vi "WBA 256 Sector (FPGA-SIM).vi"() -> ()   [LabVIEW 2013]
doc: "This is the FPGA VI for the 10-Tap 8-Bit Camera with DRAM example. This example demonstrates how to acquire images from a 10-tap, 8-bit, extended configuration, Camera Link camera and transfer the images to the host. This example supports area scan and line scan cameras for both continuous and finite acquisitions.\n\nThis example also demonstrates the use of DRAM as a frame buffer for very high speed acquisitions. Data packing and flow-control are also employed to maximize use of the available DRAM and FIFOs in terms of both memory space and performance.\n\nAdditionally, the example demonstrates the serial server, which allows third-party camera configuration utilities to communicate with the camera using the Camera Link serial interface while this VI is running."
uses:
  Common/CL Signal Mapping.ctl
  Common/CL Configuration.ctl
  FPGA/Sector/Accumulate/Sector Parameter Cluster.ctl
  <vilib>/Platform/TimedLoop/XDataNode/timing_clust.ctl
  <vilib>/Platform/TimedLoop/XDataNode/nitl_modes.ctl
  <vilib>/Platform/TimedLoop/XDataNode/wakeup.ctl
  <vilib>/rvi/Emulation/niFpgaSctlEmulationGetInTimedLoop.vi
  <vilib>/rvi/Emulation/niFpgaEmulationReportErrorSimple.vi
  <vilib>/rvi/Emulation/niFpgaGetClockAttributes.vi
  <vilib>/rvi/Emulation/niFpgaCriticalErrorInLSC.vi
  FPGA/Globals/Accumulated Sector Intensity.vi
  <vilib>/rvi/FIFO/Fifo_Resource/nirvififoEmulationGetNumberOfElementsToWriteFpgaImpl.vi
  <vilib>/rvi/DataTransferAndStorage/Container/Common/niFpgaContainerGetUniqueNameForEmu.vi
  <vilib>/rvi/interface/RandomDataEmulation/nirviRandomDataFPGAFIFO.vi
  <vilib>/rvi/interface/RandomDataEmulation/niFpgaRandomDataHandleErrors.vi
  <vilib>/rvi/FIFO/Fifo_Resource/nirvififoEmulationWriteFpgaImpl.vi
  <vilib>/rvi/FIFO/Fifo_Resource/nirvififoEmulationGetNumberOfElementsToReadFpgaImpl.vi
  <vilib>/rvi/FIFO/Fifo_Resource/nirvififoEmulationReadFpgaImpl.vi
  <vilib>/rvi/Emulation/niFpgaProcessEmulError.vi
  FPGA/Globals/Sector Parameter Global.vi
  <vilib>/rvi/eio/common/nirviEmuTemplateMethod_errors.vi
  FPGA/Globals/Pixel Location Global.vi
  <vilib>/Platform/TimedLoop/XDataNode/XDataNode.xnode
  <vilib>/rvi/DataTransferAndStorage/Container/XNode/niFpgaContainer.xnode
  <vilib>/rvi/FIFO/Fifo_Resource/nirvififoEmulationGetNumberOfElementsToWrite.vi
  <vilib>/rvi/interface/RandomDataEmulation/nirviRandomDataFpgaReadWriteTemplate.vi
  <vilib>/rvi/FIFO/Fifo_Resource/nirvififoEmulationWrite.vi
  <vilib>/rvi/FIFO/Fifo_Resource/nirvififoEmulationGetNumberOfElementsToRead.vi
  <vilib>/rvi/FIFO/Fifo_Resource/nirvififoEmulationRead.vi
  <vilib>/eio/EIONode/EIONode.xnode
  <vilib>/Platform/TimedLoop/XDataNode/XDNodeRunTimeDep.lvlib
panel:
  out "Left Sector Edge":u8
  out "Right Sector Edge":u8
  in  "Right Start Angle Duty Cycle":fxp<+,8,0>
  in  "Right End Angle Duty Cycle":fxp<+,8,0>
  in  "Left End Angle Duty Cycle":fxp<+,8,0>
  in  "Left Start Angle Duty Cycle":fxp<+,8,0>
  out "Number of Elements to Write Sector Grouping FIFO":u32
  out "Analysis Ticks":u32
  out "Target Sim TO":bool
  out "Cam Data Timeout":bool
  out "Sector FIFO Timeout":bool
  out "Host DMA Timeout":bool
  out "Number of Elements to Read Cam Data":u32
  out "Number of Elements to Write Host DMA":u32
  in  "Words per image":u32=1000
  in  "Y Resolution":u16=1000
  in  "X Resolution":u16=1000
  in  "[Average BG Intensity]":u8[](array[numeric])=[0, 0, 0, 0, 0, 0, 0, 0, 0, 0, 0, 0, 0, 0, 0, 0, 0, 0, 0, 0, 0, 0, 0, 0, 0, 0, 0, 0, 0, 0, 0, 0]
  in  "Sector Threshold":u8
  in  "# of Frames to Average":u8=1
  in  "Sector Parameters Right":T1={"Start Angle"=0.0, "End Angle"=0.4708251953125, "Inner Radius"=309, "Outter Radius"=405, "Hinge X"=685, "Hinge Y"=527, "NumWingSectors"=8}
  in  "Sector Parameters Left":T1={"Start Angle"=0.65740966796875, "End Angle"=0.99468994140625, "Inner Radius"=309, "Outter Radius"=405, "Hinge X"=464, "Hinge Y"=534, "NumWingSectors"=8}
  in  "CL Config.Configuration":T2=enum."Full"
  in  "CL Config.Signal Mapping":T3=enum."Basler 10-tap"
  in  "CL Config.Line Scan":bool
  in  "CL Config.DVAL Active High":bool=TRUE
  in  "CL Config.LVAL Active High":bool=TRUE
  in  "CL Config.FVAL Active High":bool=TRUE
  in  "CL Config.Spare Active High":bool=TRUE
  in  "Acq Control.Line Scan Height":u32
  in  "Acq Control.Frames To Acq":u32
  in  "Acq Control.Acquire":bool
  in  "Acq Control.Cancel Acq":bool
  in  "Acq Control.Ignore DVAL":bool
  in  "Acq Control.Initialize":bool
  out "Acq Status.Acq In Progress":bool
  out "Acq Status.Clocks Per Line":u32
  out "Acq Status.Frames Acq'd":u32
  out "Acq Status.Lines Per Frame":u32
  out "Acq Status.DMA Write Timeout":bool
  out "Acq Status.Initialized":bool
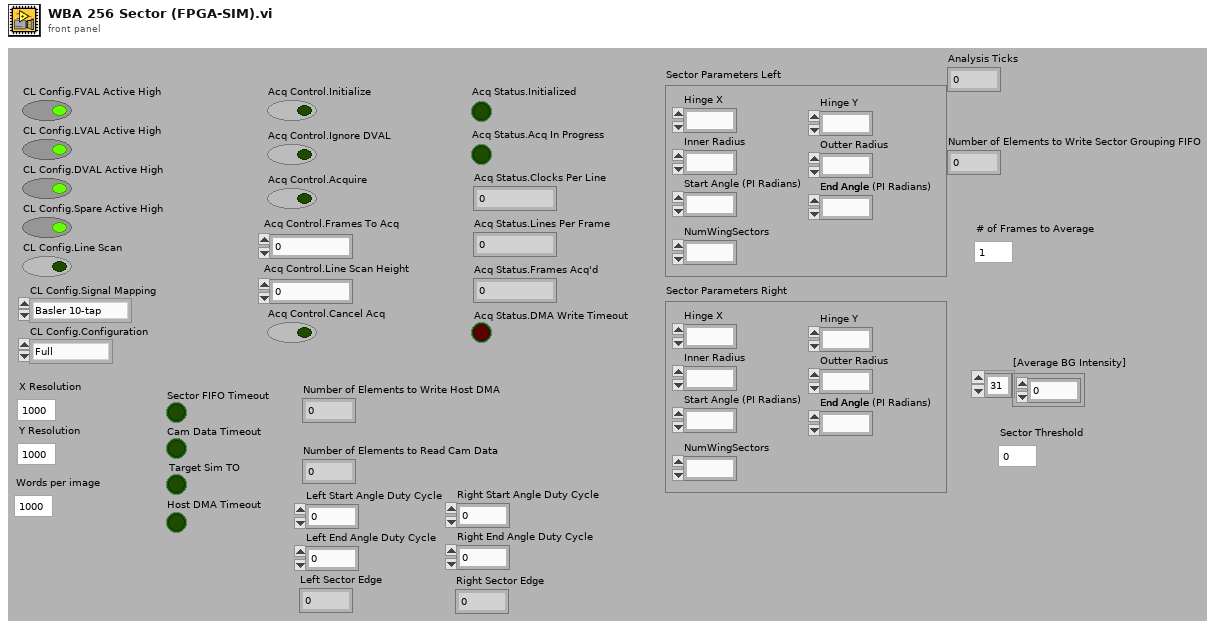
[diagram p1: front panel]
types:
  T1 = typedef "Sector Parameter Cluster.ctl" = cluster{"Start Angle":fxp<+/-,17,2>, "End Angle":fxp<+/-,17,2>, "Inner Radius":u16, "Outter Radius":u16, "Hinge X":u16, "Hinge Y":u16, "NumWingSectors":u8}
  T2 = typedef "CL Configuration.ctl" = enum8{"Base", "Medium", "Full"}
  T3 = typedef "CL Signal Mapping.ctl" = enum8{"Standard", "Basler 10-tap", "Vosskühler 10-tap"}
  T4 = typedef "XDNodeRunTimeDep.lvlib/timing_clust.ctl" = cluster{"Expected End [f-1]":u64, "Actual End [f-1]":u64, "Finished Late? [f-1]":bool, "Expected End [i-1]":u64, "Actual End [i-1]":u64, "Finished Late? [i-1]":bool, "Expected Start [i]":u64, "Actual Start [i]":u64, "Expected Start [f]":u64, "Actual Start [f]":u64, "Source Name":string, "Structure Name":string, "Period":i64, "Deadline":i64, "Offset":i64, "Start":i64, "Priority":i32, "Timeout":i32, "Mode":T5, "Wakeup Reason":T6, "Error":errorcluster, "Source Type":string, "Secondary Source Type":string, "Global End Time":u64, "Global Start Time":u64, "Frame Duration":u64, "Iteration Duration":u64, "Assigned CPU":i32, "I/O Scan Engine Mode":u32}
  T5 = typedef "XDNodeRunTimeDep.lvlib/nitl_modes.ctl" = enum32{"No Change", "Process missed periods, maintain original phase", "Discard missed periods, maintain original phase", "Process missed periods, ignore original phase", "Discard missed periods, ignore original phase"}
  T6 = typedef "XDNodeRunTimeDep.lvlib/wakeup.ctl" = enum32{"Normal", "Aborted", "Asynchronous wakeup", "Timing source error", "Timed loop error", "Timeout"}
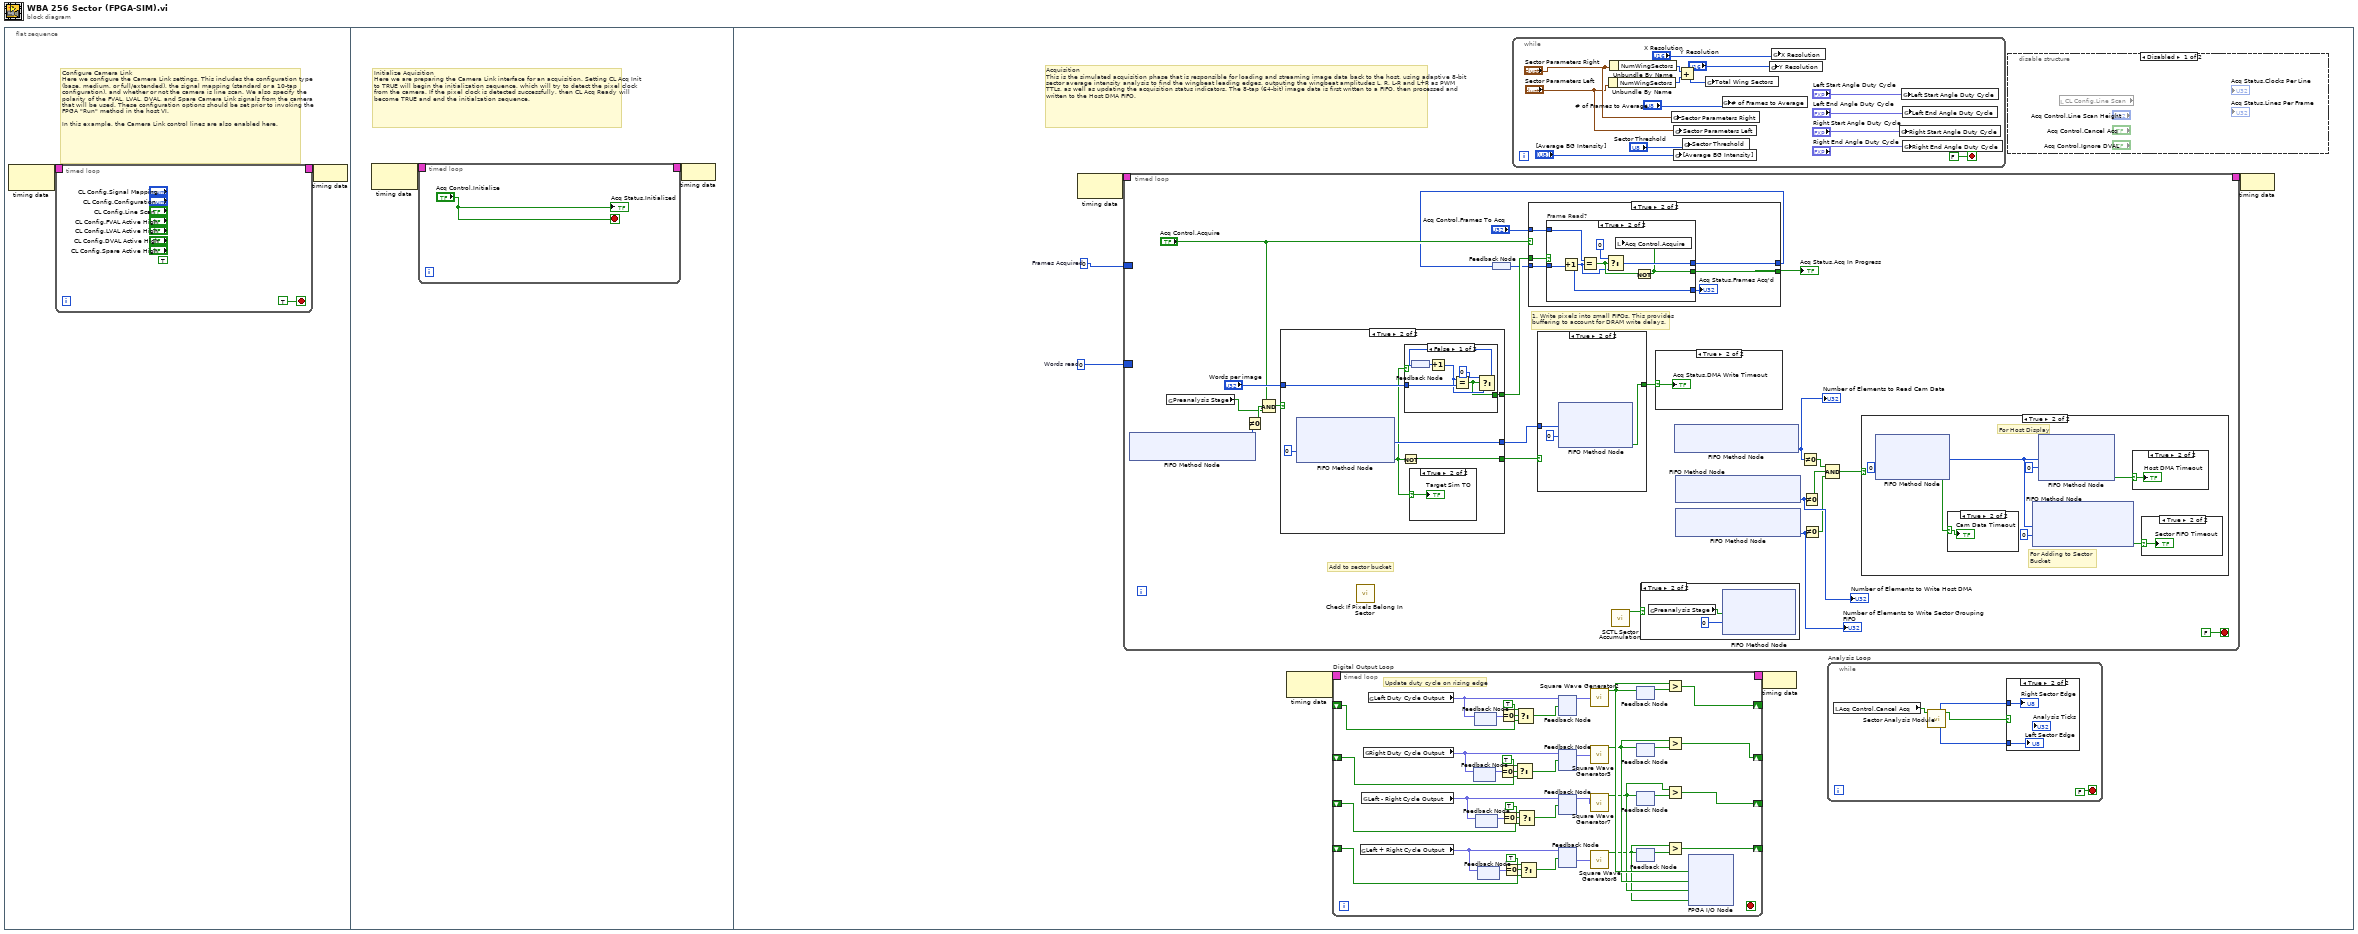
[diagram p0: block diagram]
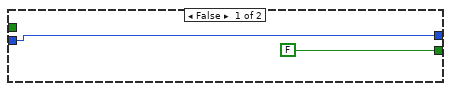
[diagram p6: hidden frame]
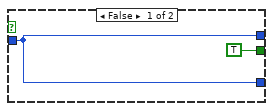
[diagram p7: hidden frame]
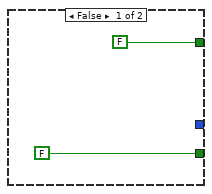
[diagram p8: hidden frame]
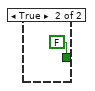
[diagram p10: hidden frame]
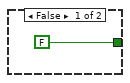
[diagram p15: hidden frame]
diagram:
  n1 = flat-sequence {
    frame #0 {
      # "Configure Camera Link\nHere we configure the Camera Link settings. This includes the configuration type (base, medium, or full/extended), the signal mapping (standard or a 10-tap configuration), and whether or not the camera is line scan. We also specify the polarity of the FVAL, LVAL, DVAL, and Spare Camera Link signals from the camera that will be used. These configuration options should be set prior to invoking the FPGA \"Run\" method in the host VI.\n\nIn this example, the Camera Link control lines are also enabled here."
      n2 = node-c288() -> (w2:T4)  [unwired: 1 in]
      n3 = timed-loop {
        timing: w2 -> [_]
        timing-out: [_] -> w1
        stop <- TRUE stop-if-true
        (unwired) TRUE ("IO Module\\CL Control Enable")
      }
      n4 = node-c288(w1) -> ()
    }
    frame #1 {
      # "Initialize Aquisition\nHere we are preparing the Camera Link interface for an acquisition. Setting CL Acq Init to TRUE will begin the initialization sequence, which will try to detect the pixel clock from the camera. If the pixel clock is detected successfully, then CL Acq Ready will become TRUE and end the initialzation sequence."
      n5 = node-c288() -> (w9:T4)  [unwired: 1 out]
      n6 = timed-loop {
        timing: w9 -> [_]
        timing-out: [_] -> w8
        stop <- "Acq Control.Initialize" stop-if-true
        "Acq Status.Initialized" <- "Acq Control.Initialize"
      }
      n7 = node-c288(w8) -> ()
    }
    frame #2 {
      w17 = u32 0  # Frames Acquired
      w18 = u32 0  # Words read
      # "Acquisition\nThis is the simulated acquisition phase that is responsible for loading and streaming image data back to the host, using adaptive 8-bit sector average intensity analysis to find the wingbeat leading edges, outputing the wingbeat amplitudes L, R, L-R and L+R as PWM TTLs, as well as updating the acquisition status indicators. The 8-tap (64-bit) image data is first written to a FIFO, then processed and written to the Host DMA FIFO."
      n8 = node-c288() -> (w20:T4)  [unwired: 1 in]
      n9 = timed-loop {
        timing: w20 -> [_]
        timing-out: [_] -> w19
        border: w18 -> [_]
        border: w17 -> [_]
        stop <- FALSE stop-if-true
        # "Add to sector bucket"
        # "1. Write pixels into small FIFOs. This provides\nbuffering to account for DRAM write delays."
        n10 = xnode ("FIFO Method Node")() -> ("Number of Elements to Write"=w88:u32)  [unwired: 1 in, 1 out]
        n11 = global read "Accumulated Sector Intensity.vi" "Preanalysis Stage"() -> (w77:bool)
        n12 = Not Equal To 0?(x=w88) -> (x != 0?=w87:bool)
        n13 = Compound Arithmetic op=AND("Acq Control.Acquire", w87, w77) -> (w95:bool)
        n14 = case shown="True" w95 {
          tunnel: [_ w127] -> w99
          tunnel: [FALSE w123] -> w97
          tunnel: "Words per image" -> [_ w125]
          tunnel: [FALSE w124] -> w84
          frame False {
          }
          frame True {
            n15 = xnode ("FIFO Method Node")("Timeout"=0) -> ("Element"=w127:u64, "Timed Out?"=w122:bool)  [unwired: 1 in, 1 out]
            n16 = Not(x=w122) -> (.not. x?=w123:bool)
            n17 = case shown="False" w122 {
              tunnel: w125 -> [w134 _]
              tunnel: [w129 FALSE] -> w124
              frame False {
                n18 = feedback #1() -> (w133:u32)
                n19 = Increment(x=w133) -> (x+1=w130:u32)
                n20 = Equal?(x=w130, y=w134) -> (x = y?=w129:bool)
                n21 = Select(t=u32 0 ("Acq Status.Frames Acq'd"), s=w129, f=w130) -> (s? t:f=w131:u32)
                n22 = feedback-in #1(w131) -> ()
              }
              frame True {
              }
            }
            n23 = case shown="True" w122 {
              selector: w122 -> [_ w128]
              frame False {
              }
              frame True {
                "Target Sim TO" <- w128
              }
            }
          }
        }
        n24 = call "Check If Pixels Belong In Sector.vi"() -> ()  [unwired: 11 in, 1 out]
        n25 = feedback #2() -> (w83:u32)
        n26 = case shown="True" "Acq Control.Acquire" {
          tunnel: w84 -> [_ w110]
          tunnel: w83 -> [w104 w109]
          tunnel: "Acq Control.Frames To Acq" -> [_ w108]
          tunnel: [w104 w107] -> w81
          tunnel: [FALSE w106] -> w80
          frame False {
          }
          frame True {
            n27 = case "Frame Read?" shown="True" w110 {
              tunnel: w109 -> [w111 w119]
              tunnel: w108 -> [_ w118]
              tunnel: [w111 w116] -> w107
              tunnel: [TRUE w114] -> w106
              tunnel: [w111 w113] -> w105
              frame False {
              }
              frame True {
                n28 = Increment(x=w119) -> (x+1=w113:u32)
                n29 = Equal?(x=w118, y=w113) -> (x = y?=w115:bool)
                n30 = Select(t=u32 0 ("Frames Acquired"), s=w115, f=w113) -> (s? t:f=w116:u32)
                n31 = Not(x=w115) -> (.not. x?=w114:bool)
                n32 = local write "Acq Control.Acquire"(w114) -> ()
              }
            }
            "Acq Status.Frames Acq'd" <- w105
          }
        }
        "Acq Status.Acq In Progress" <- w80
        n33 = feedback-in #2(w81) -> ()
        n34 = case shown="True" w97 {
          tunnel: [FALSE ("Timed Out?") w148] -> w79
          tunnel: w99 -> [_ w149]
          frame False {
          }
          frame True {
            n35 = xnode ("FIFO Method Node")("Element"=w149, "Timeout"=0) -> ("Timed Out?"=w148:bool)  [unwired: 1 in, 1 out]
          }
        }
        n36 = call "SCTL Sector Accumulation.vi"() -> ("New Data?"=w78:bool)  [unwired: 10 in, 1 out]
        n37 = case shown="True" w78 {
          frame False {
          }
          frame True {
            n38 = global read "Accumulated Sector Intensity.vi" "Preanalysis Stage"() -> (w100:bool)
            n39 = xnode ("FIFO Method Node")("Element"=w100, "Timeout"=0) -> ()  [unwired: 1 in, 2 out]
          }
        }
        n40 = case shown="True" w79 {
          selector: w79 -> [_ w102]
          frame False {
          }
          frame True {
            "Acq Status.DMA Write Timeout" <- w102
          }
        }
        n41 = xnode ("FIFO Method Node")() -> ("Number of Elements to Read"=w90:u32)  [unwired: 1 in, 1 out]
        "Number of Elements to Read Cam Data" <- w90
        n42 = xnode ("FIFO Method Node")() -> ("Number of Elements to Write"=w93:u32)  [unwired: 1 in, 1 out]
        "Number of Elements to Write Host DMA" <- w93
        n43 = xnode ("FIFO Method Node")() -> ("Number of Elements to Write"=w92:u32)  [unwired: 1 in, 1 out]
        "Number of Elements to Write Sector Grouping FIFO" <- w92
        n44 = Not Equal To 0?(x=w90) -> (x != 0?=w89:bool)
        n45 = Not Equal To 0?(x=w93) -> (x != 0?=w94:bool)
        n46 = Not Equal To 0?(x=w92) -> (x != 0?=w91:bool)
        n47 = Compound Arithmetic op=AND(w89, w94, w91) -> (w96:bool)
        n48 = case shown="True" w96 {
          frame False {
          }
          frame True {
            # "For Adding to Sector \nBucket"
            # "For Host Display"
            n49 = xnode ("FIFO Method Node")("Timeout"=0) -> ("Element"=w140:u64, "Timed Out?"=w136:bool)  [unwired: 1 in, 1 out]
            n50 = case shown="True" w136 {
              selector: w136 -> [_ w143]
              frame False {
              }
              frame True {
                "Cam Data Timeout" <- w143
              }
            }
            n51 = xnode ("FIFO Method Node")("Element"=w140, "Timeout"=0) -> ("Timed Out?"=w138:bool)  [unwired: 1 in, 1 out]
            n52 = xnode ("FIFO Method Node")("Element"=w140, "Timeout"=0) -> ("Timed Out?"=w137:bool)  [unwired: 1 in, 1 out]
            n53 = case shown="True" w137 {
              selector: w137 -> [_ w144]
              frame False {
              }
              frame True {
                "Host DMA Timeout" <- w144
              }
            }
            n54 = case shown="True" w138 {
              selector: w138 -> [_ w145]
              frame False {
              }
              frame True {
                "Sector FIFO Timeout" <- w145
              }
            }
          }
        }
      }
      n55 = node-c288() -> (w16:T4)  [unwired: 1 in]
      n56 = timed-loop "Digital Output Loop" {
        timing: w16 -> [_]
        timing-out: [_] -> w15
        shift-right: [w54] -> _
        shift-left: _ -> [w39]
        shift-right: [w53] -> _
        shift-left: _ -> [w25]
        shift-right: [w52] -> _
        shift-left: _ -> [w23]
        shift-right: [w46] -> _
        shift-left: _ -> [w21]
        stop <- _ stop-if-true
        # "Update duty cycle on rising edge"
        n57 = global read "Sector Parameter Global.vi" "Left + Right Cycle Output"() -> (w27:fxp<+,8,0>)
        n58 = global read "Sector Parameter Global.vi" "Left - Right Cycle Output"() -> (w28:fxp<+,8,0>)
        n59 = global read "Sector Parameter Global.vi" "Right Duty Cycle Output"() -> (w29:fxp<+/-,9,1>)
        n60 = global read "Sector Parameter Global.vi" "Left Duty Cycle Output"() -> (w42:fxp<+/-,9,1>)
        n61 = feedback #3() -> (w36:fxp<+/-,9,1>)  [unwired: 1 in]
        n62 = feedback-in #3(w29) -> ()
        n63 = feedback #4() -> (w41:fxp<+/-,9,1>)  [unwired: 1 in]
        n64 = feedback-in #4(w42) -> ()
        n65 = feedback #5() -> (w33:fxp<+,8,0>)  [unwired: 1 in]
        n66 = feedback-in #5(w28) -> ()
        n67 = feedback #6() -> (w30:fxp<+,8,0>)  [unwired: 1 in]
        n68 = feedback-in #6(w27) -> ()
        n69 = Equal To 0?(x=w36) -> (x = 0?=w37:bool)
        n70 = Equal To 0?(x=w41) -> (x = 0?=w43:bool)
        n71 = Equal To 0?(x=w33) -> (x = 0?=w34:bool)
        n72 = Equal To 0?(x=w30) -> (x = 0?=w31:bool)
        n73 = Select(t=TRUE, s=w37, f=w25) -> (s? t:f=w26:bool)
        n74 = Select(t=TRUE, s=w43, f=w39) -> (s? t:f=w40:bool)
        n75 = Select(t=TRUE, s=w34, f=w23) -> (s? t:f=w24:bool)
        n76 = Select(t=TRUE, s=w31, f=w21) -> (s? t:f=w22:bool)
        n77 = feedback-in #7(w42, w40) -> ()
        n78 = feedback #7() -> (w60:fxp<+/-,9,1>)  [unwired: 1 in]
        n79 = feedback #8() -> (w59:fxp<+/-,9,1>)  [unwired: 1 in]
        n80 = feedback-in #8(w29, w26) -> ()
        n81 = feedback #9() -> (w58:fxp<+,8,0>)  [unwired: 1 in]
        n82 = feedback-in #9(w28, w24) -> ()
        n83 = feedback #10() -> (w48:fxp<+,8,0>)  [unwired: 1 in]
        n84 = feedback-in #10(w27, w22) -> ()
        n85 = call "Square Wave Generator2"("duty cycle (periods)"=w60) -> ("square wave out"=w51:bool)  [unwired: 14 in]
        n86 = call "Square Wave Generator3"("duty cycle (periods)"=w59) -> ("square wave out"=w50:bool)  [unwired: 14 in]
        n87 = call "Square Wave Generator7"("duty cycle (periods)"=w58) -> ("square wave out"=w49:bool)  [unwired: 14 in]
        n88 = call "Square Wave Generator8"("duty cycle (periods)"=w48) -> ("square wave out"=w45:bool)  [unwired: 14 in]
        n89 = feedback-in #11(w51) -> ()
        n90 = feedback #11() -> (w57:bool)  [unwired: 1 in]
        n91 = feedback #12() -> (w56:bool)  [unwired: 1 in]
        n92 = feedback-in #12(w50) -> ()
        n93 = feedback #13() -> (w55:bool)  [unwired: 1 in]
        n94 = feedback-in #13(w49) -> ()
        n95 = feedback #14() -> (w47:bool)  [unwired: 1 in]
        n96 = feedback-in #14(w45) -> ()
        n97 = Greater?(x=w51, y=w57) -> (0:w54:bool)
        n98 = Greater?(x=w50, y=w56) -> (0:w53:bool)
        n99 = Greater?(x=w49, y=w55) -> (0:w52:bool)
        n100 = Greater?(x=w45, y=w47) -> (0:w46:bool)
        n101 = xnode "FPGA I/O Node"("TTL 1"=w51, "TTL 2"=w50, "TTL 3"=w49, "TTL 4"=w45) -> ()  [unwired: 4 in, 4 out]
      }
      n102 = while {
        stop <- FALSE stop-if-true
        n103 = Unbundle By Name("Sector Parameters Left") -> ("NumWingSectors"=w166:u8)
        n104 = Unbundle By Name("Sector Parameters Right") -> ("NumWingSectors"=w167:u8)
        n105 = global write "Sector Parameter Global.vi" "Sector Parameters Right"("Sector Parameters Right") -> ()
        n106 = global write "Sector Parameter Global.vi" "Sector Parameters Left"("Sector Parameters Left") -> ()
        n107 = global write "Sector Parameter Global.vi" "[Average BG Intensity]"("[Average BG Intensity]") -> ()
        n108 = Add(x=w167, y=w166) -> (x+y=w165:u8)
        n109 = global write "Sector Parameter Global.vi" "Sector Threshold"("Sector Threshold") -> ()
        n110 = global write "Accumulated Sector Intensity.vi" "Total Wing Sectors"(w165) -> ()
        n111 = global write "Pixel Location Global.vi" "# of Frames to Average"("# of Frames to Average") -> ()
        n112 = global write "Pixel Location Global.vi" "Y Resolution"("Y Resolution") -> ()
        n113 = global write "Pixel Location Global.vi" "X Resolution"("X Resolution") -> ()
        n114 = global write "Sector Parameter Global.vi" "Right Start Angle Duty Cycle"("Right Start Angle Duty Cycle") -> ()
        n115 = global write "Sector Parameter Global.vi" "Left Start Angle Duty Cycle"("Left Start Angle Duty Cycle") -> ()
        n116 = global write "Sector Parameter Global.vi" "Left End Angle Duty Cycle"("Left End Angle Duty Cycle") -> ()
        n117 = global write "Sector Parameter Global.vi" "Right End Angle Duty Cycle"("Right End Angle Duty Cycle") -> ()
      }
      n118 = node-c288(w15) -> ()
      n119 = while "Analysis Loop" {
        stop <- FALSE stop-if-true
        n120 = local read "Acq Control.Cancel Acq"() -> (w68:bool)
        n121 = call "Sector Analysis Module.vi"("Canceled?"=w68) -> ("Data"=w65:bool, "Left Sector Edge"=w66:u16, "Right Sector Edge"=w67:u16)  [unwired: 7 in, 1 out]
        n122 = case shown="True" w65 {
          tunnel: w67 -> [_ w71]
          tunnel: w66 -> [_ w70]
          frame False {
          }
          frame True {
            "Right Sector Edge" <- w71
            "Left Sector Edge" <- w70
          }
        }
      }
      n123 = disable-structure shown="Disabled" {
        frame Disabled {
          n124 = local read "CL Config.Line Scan"() -> (w74:bool)
        }
        frame Enabled {
        }
      }
      n125 = node-c288(w19) -> ()
    }
  }
